vi "RunRawREPL.vi"() -> ()   [LabVIEW 2016]
panel:
  out "Console Out":string
  in  "VISA":refnum<visa-resource-name>
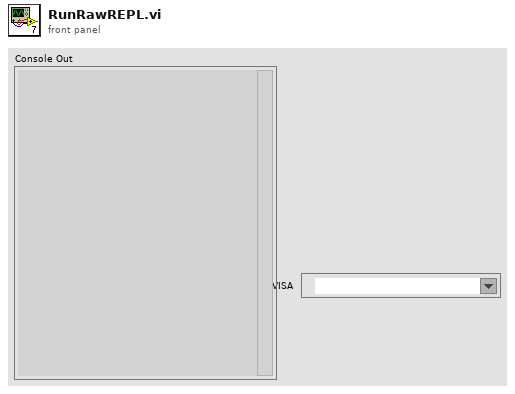
[diagram p1: front panel]
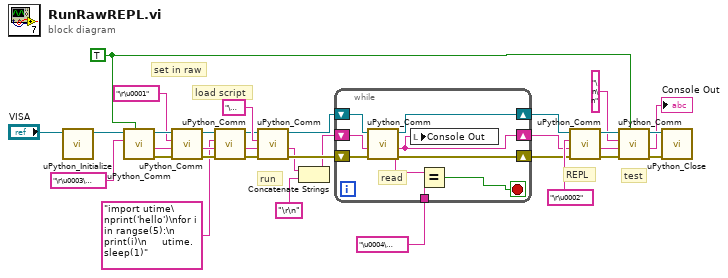
[diagram p0: block diagram]
diagram:
  w11 = TRUE ("Wait for Reply?")
  # "test"
  # "REPL"
  # "run"
  # "load script"
  # "set in raw"
  n1 = call "uPython_Initialize.vi"("VISA Refnum in"="VISA") -> ("VISA Refnum out"=w32:refnum<visa-resource-name>)  [unwired: 9 in, 1 out]
  n2 = call "uPython_Comm.vi"("Wait for Reply?"=w11, "Script"="\r\u0003\u0003", "VISA Refnum in"=w32) -> ("error out"=w29:errorcluster, "Console Out"=w27:string, "VISA out"=w30:refnum<visa-resource-name>)  [unwired: 4 in, 2 out]
  n3 = call "uPython_Comm.vi"("error in (no error)"=w29, "Console In"=w27, "Script"="\r\u0001", "VISA Refnum in"=w30) -> ("error out"=w17:errorcluster, "Console Out"=w16:string, "VISA out"=w18:refnum<visa-resource-name>)  [unwired: 3 in, 2 out]
  n4 = call "uPython_Comm.vi"("error in (no error)"=w17, "Console In"=w16, "Script"="import utime\nprint('hello')\nfor i in rangse(5):\n     print(i)\n     utime.sleep(1)", "VISA Refnum in"=w18) -> ("error out"=w12:errorcluster, "Console Out"=w10:string, "VISA out"=w13:refnum<visa-resource-name>)  [unwired: 3 in, 2 out]
  n5 = call "uPython_Comm.vi"("error in (no error)"=w12, "Console In"=w10, "Script"="\u0004", "VISA Refnum in"=w13) -> ("error out"=w9:errorcluster, "Console Out"=w3:string, "VISA out"=w8:refnum<visa-resource-name>)  [unwired: 3 in, 2 out]
  n6 = Concatenate Strings(w3, "\r\n" ("Script")) -> (w1:string)
  n7 = while {
    shift-right: [w39] -> w6
    shift-left: w9 -> [w42]
    shift-right: [w40] -> w7
    shift-left: w8 -> [w41]
    shift-right: [w37] -> w5
    shift-left: w1 -> [w38]
    tunnel: "\u0004\u0004>" ("Script") -> [w35]
    stop <- w34 stop-if-true
    # "read"
    n8 = call "uPython_Comm.vi"("error in (no error)"=w42, "Console In"=w38, "VISA Refnum in"=w41) -> ("error out"=w39:errorcluster, "Console Out"=w37:string, "Buffer"=w36:string, "VISA out"=w40:refnum<visa-resource-name>)  [unwired: 4 in, 1 out]
    n9 = local write "Console Out"(w37) -> ()
    n10 = Equal?(x=w36, y=w35) -> (x = y?=w34:bool)
  }
  n11 = call "uPython_Comm.vi"("error in (no error)"=w6, "Console In"=w5, "Script"="\r\u0002", "VISA Refnum in"=w7) -> ("error out"=w25:errorcluster, "Console Out"=w24:string, "VISA out"=w23:refnum<visa-resource-name>)  [unwired: 3 in, 2 out]
  n12 = call "uPython_Comm.vi"("Wait for Reply?"=w11, "error in (no error)"=w25, "Console In"=w24, "Script"="\n\n", "VISA Refnum in"=w23) -> ("error out"=w22:errorcluster, "Console Out"=→"Console Out":string, "VISA out"=w21:refnum<visa-resource-name>)  [unwired: 2 in, 2 out]
  n13 = call "uPython_Close.vi"("error in"=w22, "VISA  in"=w21) -> ()  [unwired: 8 in, 2 out]
